vi "PH_OceanOpticsSpectrometer.ProcPeriodic.vi"(0 "i ref in":refnum<vi>, 3 "ms timeout (100)":i32=100, 5 "error in (no error)":errorcluster) -> (14 "i ref out":refnum<vi>, 17 "timed out":bool, 19 "error out":errorcluster)   [LabVIEW 2014, in "PH_OceanOpticsSpectrometer.lvlib"]
doc: "This method serves to periodically do things like reading values from the HW. Methods that should be executed periodically should be called from THIS methode. Add code here."
uses:
  PH_OceanOpticsSpectrometer.lvlib
  PH_StatusHandler/PH_StatusHandler.lvlib
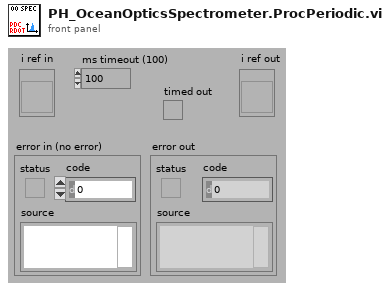
[diagram p1: front panel]
types:
  T1 = typedef "PH_StatusHandler.lvlib/PH_StatusHandler.Status.ctl" = i16
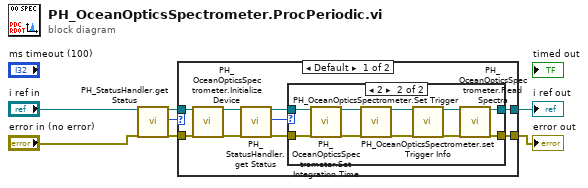
[diagram p0: block diagram]
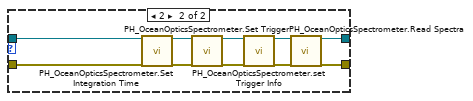
[diagram p3: hidden frame]
diagram:
  n1 = call "PH_StatusHandler.get Status.vi"("VI in"="i ref in", "error in"="error in (no error)") -> ("VI out"=w2:refnum<vi>, "Status"=w1:T1, "error out"=w3:errorcluster)  [unwired: 15 in]
  n2 = case shown="Default" w1 {
    tunnel: [w16 w38] -> w7
    tunnel: [w15 w37] -> w6
    tunnel: w3 -> [w14 w35]
    tunnel: w2 -> [w13 w36]
    frame Default {
      n3 = call "PH_OceanOpticsSpectrometer.Initialize Device.vi"("i ref in"=w13, "error in (no error)"=w14) -> ("i ref out"=w10:refnum<vi>, "error out"=w12:errorcluster)  [unwired: 16 in]
      n4 = call "PH_StatusHandler.get Status.vi"("VI in"=w10, "error in"=w12) -> ("VI out"=w9:refnum<vi>, "Status"=w8:T1, "error out"=w11:errorcluster)  [unwired: 15 in]
      n5 = case shown="2" w8 {
        tunnel: [w18 w28] -> w16
        tunnel: [w17 w27] -> w15
        tunnel: w11 -> [w17 w20]
        tunnel: w9 -> [w18 w19]
        frame Default {
        }
        frame 2 {
          n6 = call "PH_OceanOpticsSpectrometer.Set Integration Time.vi"("i ref in"=w19, "error in (no error)"=w20) -> ("i ref out"=w25:refnum<vi>, "error out"=w26:errorcluster)  [unwired: 16 in]
          n7 = call "PH_OceanOpticsSpectrometer.Set Trigger.vi"("i ref in"=w25, "error in (no error)"=w26) -> ("i ref out"=w22:refnum<vi>, "error out"=w24:errorcluster)  [unwired: 16 in]
          n8 = call "PH_OceanOpticsSpectrometer.set Trigger Info.vi"("i ref in"=w22, "error in (no error)"=w24) -> ("i ref out"=w21:refnum<vi>, "error out"=w23:errorcluster)  [unwired: 16 in]
          n9 = call "PH_OceanOpticsSpectrometer.Read Spectra.vi"("i ref in"=w21, "error in (no error)"=w23) -> ("i ref out"=w28:refnum<vi>, "error out"=w27:errorcluster)  [unwired: 16 in]
        }
      }
    }
    frame 2 {
      n10 = call "PH_OceanOpticsSpectrometer.Set Integration Time.vi"("i ref in"=w36, "error in (no error)"=w35) -> ("i ref out"=w33:refnum<vi>, "error out"=w34:errorcluster)  [unwired: 16 in]
      n11 = call "PH_OceanOpticsSpectrometer.Set Trigger.vi"("i ref in"=w33, "error in (no error)"=w34) -> ("i ref out"=w30:refnum<vi>, "error out"=w32:errorcluster)  [unwired: 16 in]
      n12 = call "PH_OceanOpticsSpectrometer.set Trigger Info.vi"("i ref in"=w30, "error in (no error)"=w32) -> ("i ref out"=w29:refnum<vi>, "error out"=w31:errorcluster)  [unwired: 16 in]
      n13 = call "PH_OceanOpticsSpectrometer.Read Spectra.vi"("i ref in"=w29, "error in (no error)"=w31) -> ("i ref out"=w38:refnum<vi>, "error out"=w37:errorcluster)  [unwired: 16 in]
    }
  }
  "error out" <- w6
  "i ref out" <- w7
